vi "temp chart calculations.vi"(0 "temp in":dbl format="%.2f", 7 "Control Parameters":T1={"Setpoint"=50.0, "Control bandwidth"=4.0, "Settle bandwidth"=1.0, "Integral time"=30.0, "Int\non"=TRUE, "Derivative time"=0.5, "Der\non"=TRUE, "Settle time"=200.0} {"Settle time" format="%.2f"; "Derivative time" format="%.2f"; "Integral time" format="%.2f"; "Settle bandwidth" format="%.2f"; "Control bandwidth" format="%.2f"; "Setpoint" format="%.2f"}, 9 "Temperature History in":refnum<vi>, 11 "norm power in":dbl format="%.2f", 13 "Mode":enum16{"Expanded", "Shrunk"}(ring)) -> (4 "Temperature History":T3 {"?" format="%.2f"; "?" format="%.2f"; "?" format="%.2f"; "?" format="%.2f"; "?" format="%.2f"; "?" format="%.2f"; "temp out" format="%.2f"}, 8 "range indicators":T2={"In control band"=TRUE, "In settle band"=TRUE, "under range"=TRUE, "over range"=TRUE}, 10 "Temperature History out":refnum<vi>)   [LabVIEW 2014]
doc: "This subvi does various calculations for the temperature controller display\n\nPaul K Dixon\nPhysics 350\nPaul K Dixon"
uses:
  typedefs/status indicator.ctl
  typedefs/control parameters.ctl
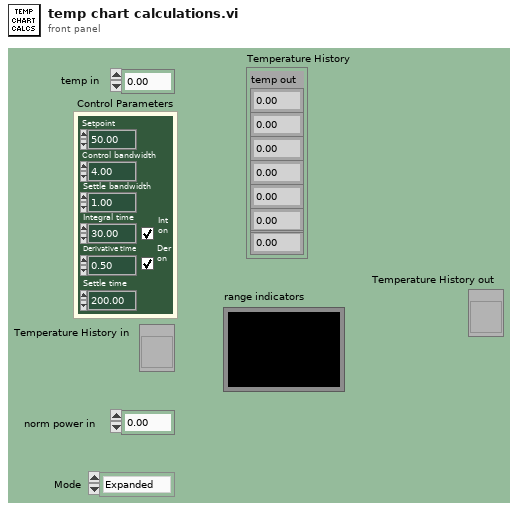
[diagram p1: front panel]
types:
  T1 = typedef "control parameters.ctl" = cluster{"Setpoint":dbl, "Control bandwidth":dbl, "Settle bandwidth":dbl, "Integral time":dbl, "Int\non":bool, "Derivative time":dbl, "Der\non":bool, "Settle time":dbl}
  T2 = typedef "status indicator.ctl" = cluster{"In control band":bool, "In settle band":bool, "under range":bool, "over range":bool}
  T3 = cluster{"temp out":dbl, dbl, dbl, dbl, dbl, dbl, dbl}
  T4 = cluster{"temp in":dbl, "Setpoint":dbl, "THC":dbl, "TLC":dbl, "THS":dbl, "TLS":dbl, dbl}
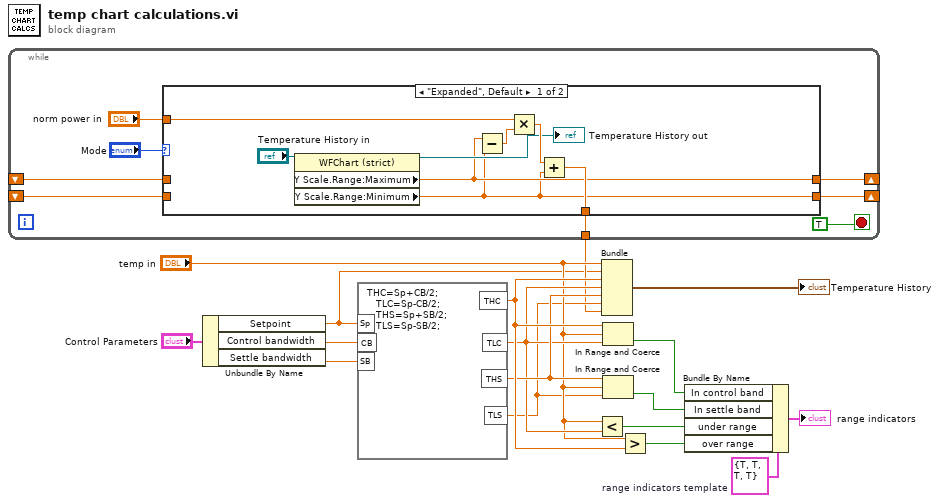
[diagram p0: block diagram]
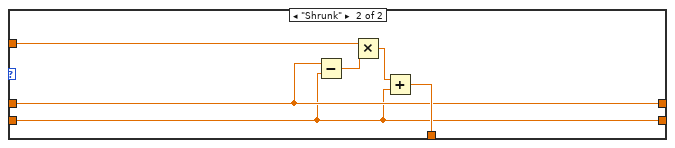
[diagram p2: hidden frame]
diagram:
  w10 = T2 {"In control band"=TRUE, "In settle band"=TRUE, "under range"=TRUE, "over range"=TRUE}  # range indicators template
  n1 = while {
    tunnel: [w25] -> w11
    shift-right: [w21] -> _
    shift-left: _ -> [w19]
    shift-right: [w20] -> _
    shift-left: _ -> [w18]
    stop <- TRUE stop-if-true
    n2 = case shown="\"Expanded\", Default" "Mode" {
      tunnel: [w32 w38] -> w25
      tunnel: "norm power in" -> [w28 w36]
      tunnel: [w27 w35] -> w21
      tunnel: [w26 w34] -> w20
      tunnel: w19 -> [_ w35]
      tunnel: w18 -> [_ w34]
      frame "Expanded", Default {
        n3 = property class="WFChart (strict)"(reference="Temperature History in") -> (reference out=→"Temperature History out":refnum<vi>, "Y Scale.Range:Maximum"=w27:dbl, "Y Scale.Range:Minimum"=w26:dbl)  [unwired: 1 in, 1 out]
        n4 = Subtract(x=w27, y=w26) -> (x-y=w31:dbl)
        n5 = Multiply(x=w28, y=w31) -> (x*y=w33:dbl)
        n6 = Add(x=w33, y=w26) -> (x+y=w32:dbl)
      }
      frame "Shrunk" {
        n7 = Subtract(x=w35, y=w34) -> (x-y=w37:dbl)
        n8 = Multiply(x=w36, y=w37) -> (x*y=w39:dbl)
        n9 = Add(x=w39, y=w34) -> (x+y=w38:dbl)
      }
    }
  }
  n10 = Unbundle By Name("Control Parameters") -> ("Setpoint"=w3:dbl, "Control bandwidth"=w2:dbl, "Settle bandwidth"=w1:dbl)
  n11 = formula code="THC=Sp+CB/2;\n   TLC=Sp-CB/2;\n   THS=Sp+SB/2;\n   TLS=Sp-SB/2;"("Sp"=w3, "CB"=w2, "SB"=w1) -> ("THC"=w17:dbl, "TLC"=w15:dbl, "THS"=w16:dbl, "TLS"=w12:dbl)
  n12 = Less?(x="temp in", y=w15) -> (x < y?=w6:bool)
  n13 = Bundle("temp in"="temp in", "Setpoint"=w3, "THC"=w17, "TLC"=w15, "THS"=w16, "TLS"=w12, w11) -> (→"Temperature History":T4)  [unwired: 1 out]
  n14 = In Range and Coerce(upper limit=w17, x="temp in", lower limit=w15) -> (In Range?=w8:bool)  [unwired: 1 out]
  n15 = In Range and Coerce(upper limit=w16, x="temp in", lower limit=w12) -> (In Range?=w5:bool)  [unwired: 1 out]
  n16 = Greater?(x="temp in", y=w17) -> (0:w7:bool)
  n17 = Bundle By Name(cluster=w10, "In control band"=w8, "In settle band"=w5, "under range"=w6, "over range"=w7) -> (→"range indicators":T2)
